vi "subvi_analyser_moving.vi"(9 "Current Angles":cluster{"Analyser 1":i32, "Analyser 2":i32}, 11 "Set Angles":cluster{"Analyser 1":i32, "Analyser 2":i32}) -> (3 "Analysers Moving?":T1)   [LabVIEW 2014]
doc: "Subvi to compare Current Angles and Set Angles of analysers and return\na cluster of bools denoting whether the analysers should move.\nManish Patel\nLast date edited: 15/08/2019"
panel:
  # "INPUTS"
  # "OUTPUTS"
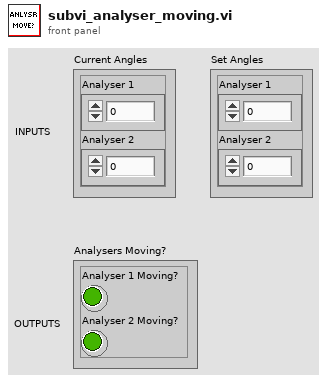
[diagram p1: front panel]
types:
  T1 = cluster{"Analyser 1 Moving?":bool, "Analyser 2 Moving?":bool}
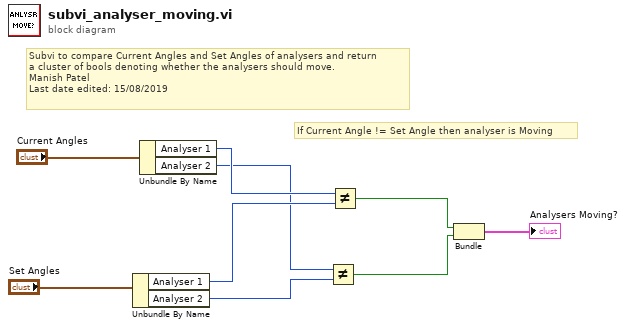
[diagram p0: block diagram]
diagram:
  # "Subvi to compare Current Angles and Set Angles of analysers and return\na cluster of bools denoting whether the analysers should move.\nManish Patel\nLast date edited: 15/08/2019"
  # "If Current Angle != Set Angle then analyser is Moving"
  n1 = Unbundle By Name("Set Angles") -> ("Analyser 1"=w6:i32, "Analyser 2"=w4:i32)
  n2 = Unbundle By Name("Current Angles") -> ("Analyser 1"=w7:i32, "Analyser 2"=w5:i32)
  n3 = Not Equal?(x=w5, y=w4) -> (x != y?=w1:bool)
  n4 = Not Equal?(x=w7, y=w6) -> (x != y?=w2:bool)
  n5 = Bundle(w2, w1) -> (→"Analysers Moving?":cluster{bool, bool})  [unwired: 1 in]
